vi "Move In Next Page.vi"(8 "error in (no error)":errorcluster, 11 "Sensor View in":refnum<class "Sensor View.lvclass">) -> (0 "error out":errorcluster, 3 "Sensor View out":refnum<class "Sensor View.lvclass">)   [LabVIEW 2013, in "Sensor View.lvlib" / "Sensor View.lvclass"]
uses:
  Sensor View.lvclass
  Sensor View.lvclass/Sensor View.ctl
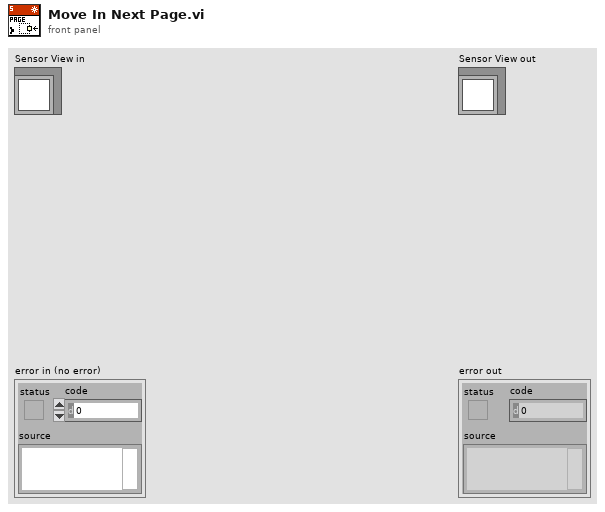
[diagram p1: front panel]
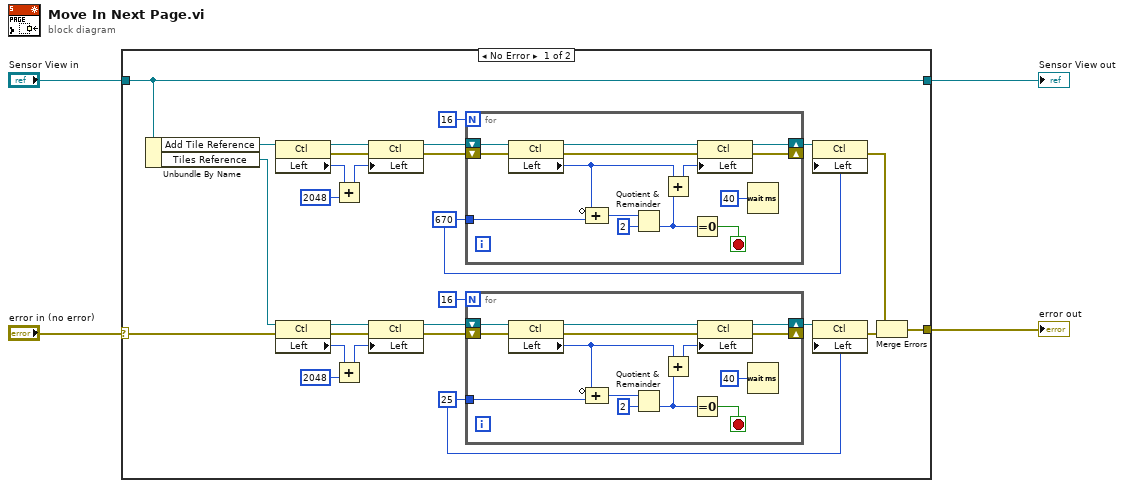
[diagram p0: block diagram]
diagram:
  n1 = case shown="No Error" "error in (no error)" {
    selector: "error in (no error)" -> [w31 w61]
    tunnel: [w30 w61] -> w3
    tunnel: "Sensor View in" -> [w5 w60]
    tunnel: [w5 w60] -> w1
    frame No Error {
      w21 = 25 ("Splitter Position")
      w22 = 670 ("Splitter Position")
      n2 = Unbundle By Name(w5) -> ("Add Tile Reference"=w27:refnum<vi>, "Tiles Reference"=w14:refnum<vi>)
      n3 = property class="Ctl"(reference=w27) -> (reference out=w29:refnum<vi>, error out=w11:errorcluster, "Left"=w26:i32)  [unwired: 1 in]
      n4 = property class="Ctl"(reference=w14, error in=w31) -> (reference out=w15:refnum<vi>, error out=w12:errorcluster, "Left"=w17:i32)
      n5 = Add(x=w26, y=2048 ("Position:Left")) -> (x+y=w25:i32)
      n6 = Add(x=w17, y=2048 ("Position:Left")) -> (x+y=w18:i32)
      n7 = property class="Ctl"(reference=w29, error in=w11, "Left"=w25) -> (reference out=w24:refnum<vi>, error out=w10:errorcluster)
      n8 = property class="Ctl"(reference=w15, error in=w12, "Left"=w18) -> (reference out=w19:refnum<vi>, error out=w13:errorcluster)
      n9 = for {
        N: 16 -> [_]
        shift-right: [w57] -> w23
        shift-left: w24 -> [w59]
        shift-right: [w50] -> _
        shift-left: w10 -> [w58]
        tunnel: w22 -> [w46]
        stop <- w49 stop-if-true
        n10 = property class="Ctl"(reference=w59, error in=w58) -> (reference out=w55:refnum<vi>, error out=w56:errorcluster, "Left"=w47:i32)
        n11 = Compound Arithmetic op=ADD(invert w47, w46) -> (w53:i32)
        n12 = Quotient & Remainder(x=w53, y=2) -> (floor(x/y)=w51:i32)  [unwired: 1 out]
        n13 = Add(x=w47, y=w51) -> (x+y=w54:i32)
        n14 = Equal To 0?(x=w51) -> (x = 0?=w49:bool)
        n15 = property class="Ctl"(reference=w55, error in=w56, "Left"=w54) -> (reference out=w57:refnum<vi>, error out=w50:errorcluster)
        n16 = Wait (ms)(milliseconds to wait=u32 40) -> ()  [unwired: 1 out]
      }
      n17 = for {
        N: 16 -> [_]
        shift-right: [w43] -> w20
        shift-left: w19 -> [w45]
        shift-right: [w36] -> _
        shift-left: w13 -> [w44]
        tunnel: w21 -> [w32]
        stop <- w35 stop-if-true
        n18 = property class="Ctl"(reference=w45, error in=w44) -> (reference out=w41:refnum<vi>, error out=w42:errorcluster, "Left"=w33:i32)
        n19 = Compound Arithmetic op=ADD(invert w33, w32) -> (w39:i32)
        n20 = Quotient & Remainder(x=w39, y=2) -> (floor(x/y)=w37:i32)  [unwired: 1 out]
        n21 = Add(x=w33, y=w37) -> (x+y=w40:i32)
        n22 = Equal To 0?(x=w37) -> (x = 0?=w35:bool)
        n23 = property class="Ctl"(reference=w41, error in=w42, "Left"=w40) -> (reference out=w43:refnum<vi>, error out=w36:errorcluster)
        n24 = Wait (ms)(milliseconds to wait=u32 40) -> ()  [unwired: 1 out]
      }
      n25 = property class="Ctl"(reference=w23, "Left"=w22) -> (error out=w8:errorcluster)  [unwired: 1 in, 1 out]
      n26 = property class="Ctl"(reference=w20, "Left"=w21) -> (error out=w9:errorcluster)  [unwired: 1 in, 1 out]
      n27 = Merge Errors(w8, w9) -> (w30:errorcluster)
    }
    frame Error {
    }
  }
  "error out" <- w3
  "Sensor View out" <- w1
